vi "Handle getAll.vi"(8 "error in (no error)":errorcluster, 11 "Inst.TC in":refnum<class "Inst.TC.lvclass">) -> (0 "error out":errorcluster, 2 "getAll":variant, 3 "Inst.TC out":refnum<class "Inst.TC.lvclass">)   [LabVIEW 2019, in "Inst.TC.lvclass"]
uses:
  Inst.TC.lvclass
  Inst.TC.lvclass/Inst.TC.ctl
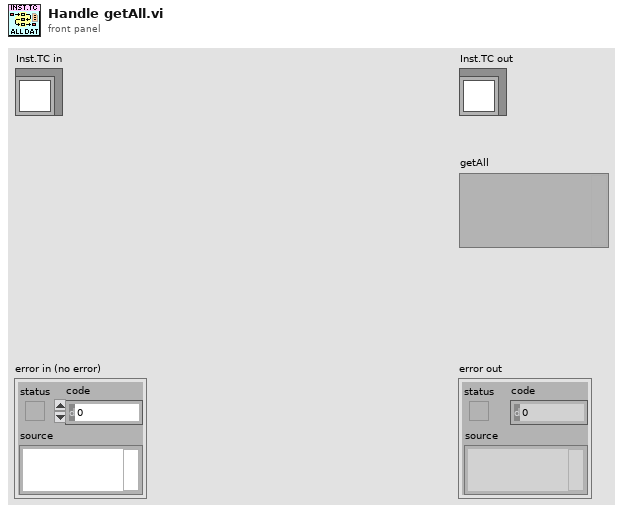
[diagram p1: front panel]
types:
  T1 = typedef "Inst.TC.lvclass/Inst.TC.getAll--Cluster.ctl" = cluster{"R":dbl[], "T":dbl[], "I":dbl[], "AVS Names":string, "Calibrations":string}
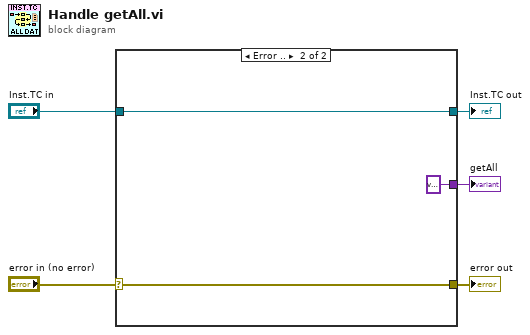
[diagram p0: block diagram]
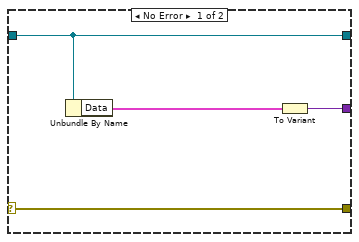
[diagram p2: hidden frame]
diagram:
  n1 = case shown="Error .." "error in (no error)" {
    selector: "error in (no error)" -> [w7 w12]
    tunnel: "Inst.TC in" -> [w6 w11]
    tunnel: [w8 variant ("Variant")] -> w4
    tunnel: [w7 w12] -> w2
    tunnel: [w6 w11] -> w1
    frame No Error {
      n2 = Unbundle By Name(w6) -> ("Data"=w9:T1)
      n3 = To Variant(anything=w9) -> (Variant=w8:variant)
    }
    frame Error {
    }
  }
  "error out" <- w2
  "Inst.TC out" <- w1
  "getAll" <- w4
